vi "Launch.vi"(8 "error in (no error)":errorcluster, 11 "Thread in":refnum<class "Thread.lvclass">) -> (0 "error out":errorcluster, 3 "Thread out":refnum<class "Thread.lvclass">)   [LabVIEW 2017, in "DSF Core.lvlib" / "Thread.lvclass"]
uses:
  Thread.lvclass
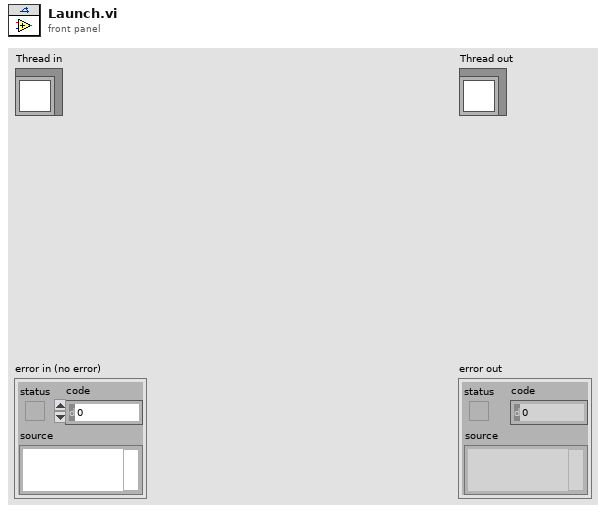
[diagram p1: front panel]
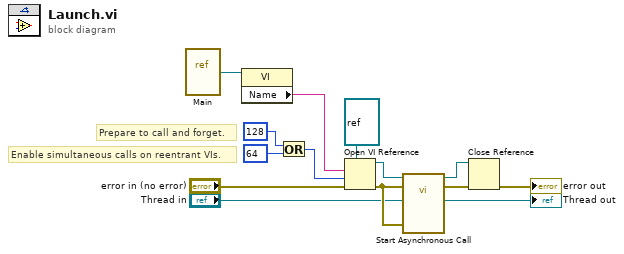
[diagram p0: block diagram]
diagram:
  # "Prepare to call and forget."
  # "Enable simultaneous calls on reentrant VIs."
  n1 = vi-ref "Main.vi"() -> (w5:refnum<vi>)
  n2 = property class="VI"(reference=w5) -> ("Name"=w1:string)  [unwired: 1 in, 2 out]
  n3 = Or(x=128 ("options"), y=64 ("options")) -> (x .or. y?=w6:i32)
  n4 = Open VI Reference(type specifier VI Refnum (for type only)=refnum<vi> refnum, vi path=w1, options=w6, error in (no error)="error in (no error)") -> (vi reference=w11:refnum<vi>, error out=w13:errorcluster)  [unwired: 2 in]
  n5 = call-by-ref "Start Asynchronous Call"(reference=w11, error in=w13, 8:"error in (no error)"=w13, "Thread in"="Thread in") -> (reference out=w9:refnum<vi>, error out=w10:errorcluster)  [unwired: 8 in, 2 out]
  n6 = Close Reference(reference=w9, error in (no error)=w10) -> (error out=→"error out":errorcluster)
  "Thread out" <- "Thread in"
